vi "AutoMod.vi"() -> ()   [LabVIEW 2016]
panel:
  out "Auto Mod indic":dbl
  in  "Auto Mod contr":dbl
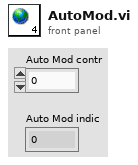
[diagram p1: front panel]
diagram:
